vi "denso gripper.vi"() -> ()   [LabVIEW 2016]
uses:
  <vilib>/DENSO Robotics/DENSO Robot Library/_DNWA/DENSO RC8 Motion interpolation Enumeration.ctl
  <vilib>/DENSO Robotics/DENSO Robot Library/_DNWA/DENSO RC8 Motion Option Cluster.ctl
  <vilib>/DigiMetrix/Schunk WSG Library/Schunk WSG library.lvlib
  <vilib>/DENSO Robotics/DENSO Robot Library/_DNWA/RC8 Library.lvlib
panel:
  out "element":dbl
  out "array":dbl[][](array[numeric])
  in  "IP address":string="192.168.1.140"
  out "error out":errorcluster
  out "?":string
  in  "Motion interpolation":T1=1 items=["P"=1, "L"=2, "C"=3]
  out "success":bool
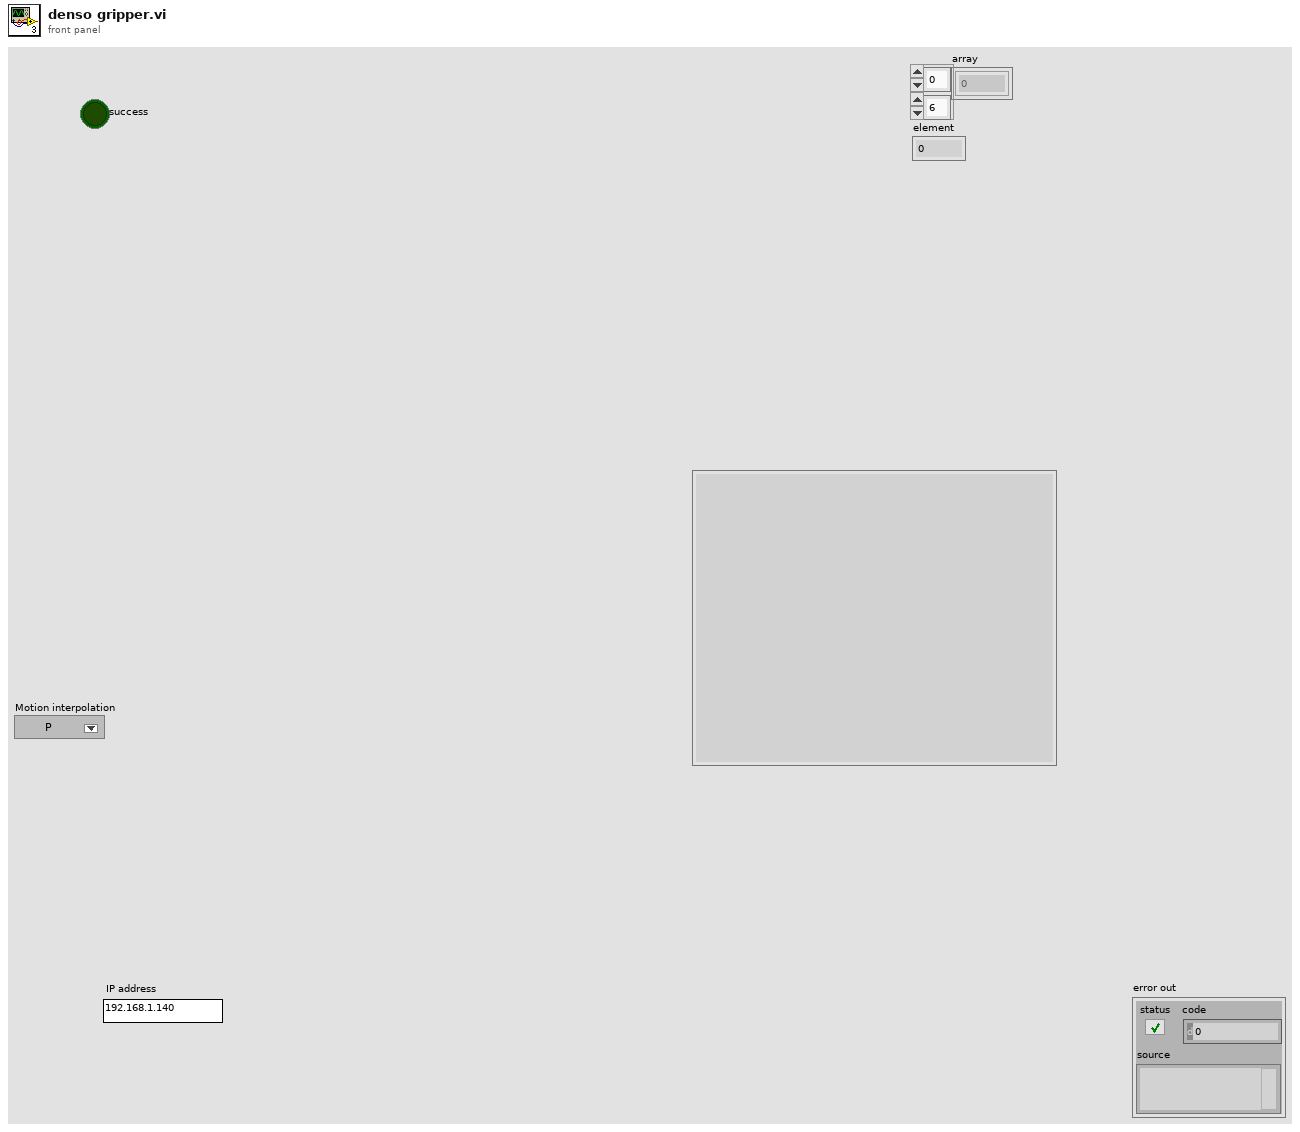
[diagram p1: front panel]
types:
  T1 = typedef "DENSO b-CAP Library.lvlib/RC8 Library.lvlib/DENSO RC8 Motion interpolation Enumeration.ctl" = i32
  T2 = typedef "DENSO b-CAP Library.lvlib/RC8 Library.lvlib/DENSO RC8 Motion Option Cluster.ctl" = cluster{"Asynchronous execution option":bool, "[SPEED=n][,ACCEL=n][,DECEL=n][,TIME=n]":string}
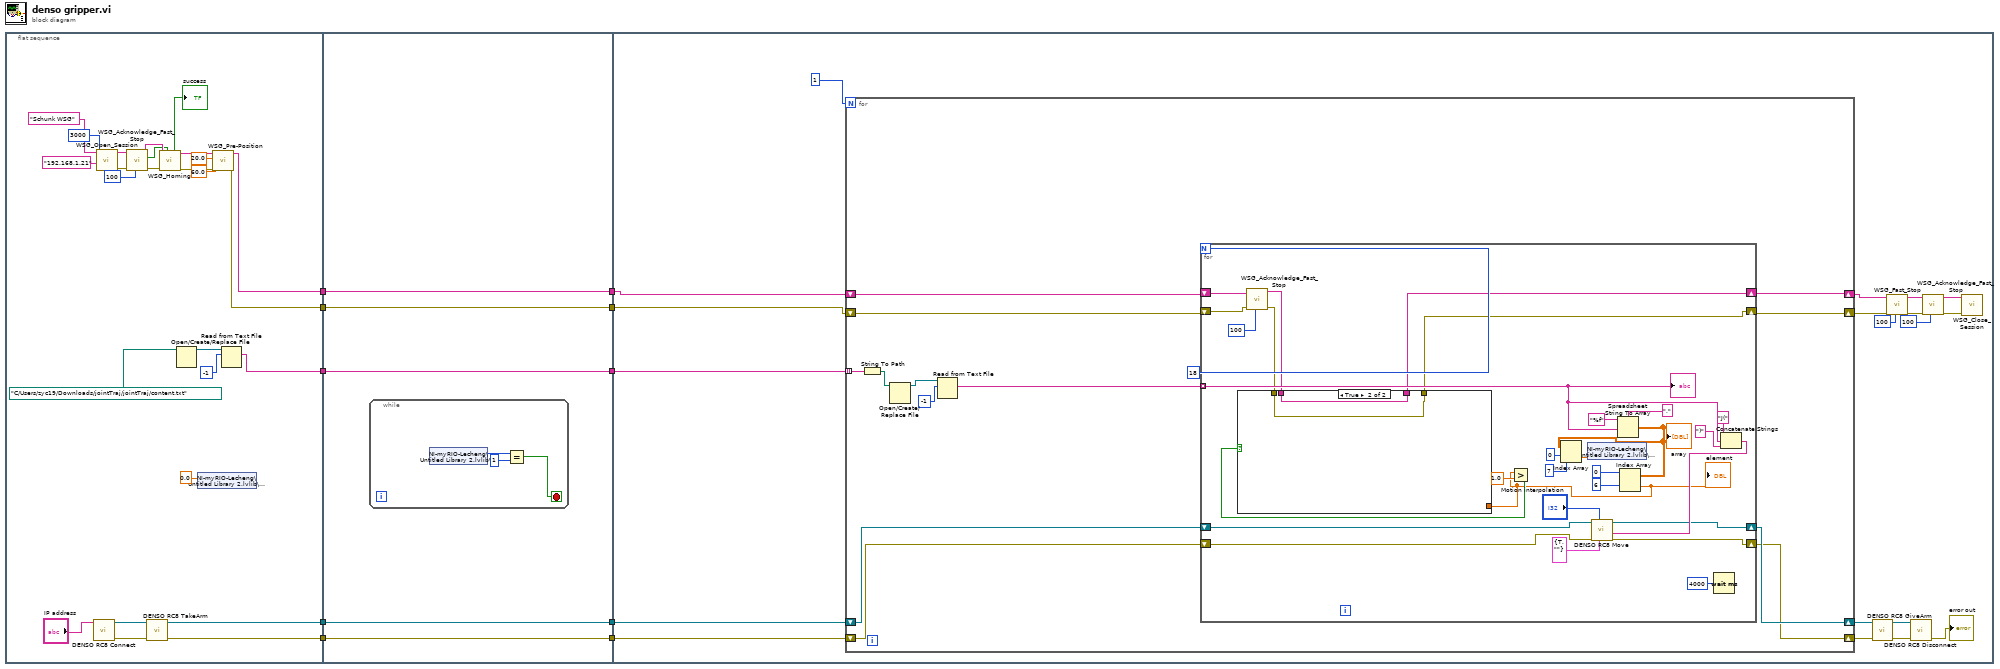
[diagram p0: block diagram]
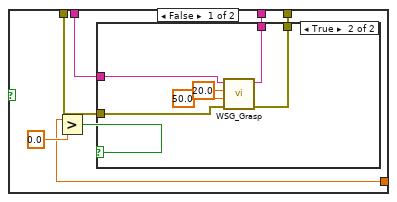
[diagram p2: hidden frame]
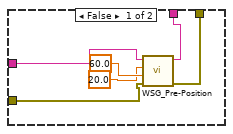
[diagram p3: hidden frame]
diagram:
  n1 = flat-sequence {
    tunnel: [w30] -> w10
    tunnel: [w29] -> w8
    tunnel: [w28] -> w5
    tunnel: [w13] -> w3
    tunnel: [w12] -> w2
    tunnel: w10 -> [w41]
    tunnel: [w41] -> w9
    tunnel: w8 -> [w40]
    tunnel: [w40] -> w7
    tunnel: [w39] -> w6
    tunnel: w5 -> [w39]
    tunnel: [w38] -> w4
    tunnel: w3 -> [w38]
    tunnel: w2 -> [w37]
    tunnel: [w37] -> w1
    tunnel: w9 -> [w52]
    tunnel: w7 -> [w51]
    tunnel: w6 -> [w50]
    tunnel: w4 -> [w49]
    tunnel: w1 -> [w48]
    frame #0 {
      n2 = call <vilib>:"DENSO RC8 Connect.vi"("IP address"="IP address") -> ("error out"=w33:errorcluster, "DENSO b-CAP Client out"=w32:refnum<class "DENSO b-CAP Client.lvclass">)  [unwired: 9 in]
      n3 = call <vilib>:"WSG_Open_Session.vi"("ip address"="192.168.1.21", "port"=u16 3000, "wsg session name"="Schunk WSG") -> ("error out"=w27:errorcluster, "wsg session name*"=w26:string)  [unwired: 7 in]
      n4 = call <vilib>:"WSG_Acknowledge_Fast_Stop.vi"("timeout"=100, "error in (no error)"=w27, "wsg session name"=w26) -> ("error out"=w22:errorcluster, "success"=w23:bool, "wsg session name*"=w24:string)  [unwired: 5 in, 1 out]
      n5 = call <vilib>:"DENSO RC8 TakeArm.vi"("error in (no error)"=w33, "DENSO b-CAP Client in"=w32) -> ("error out"=w29:errorcluster, "DENSO b-CAP Client out"=w30:refnum<class "DENSO b-CAP Client.lvclass">)  [unwired: 8 in]
      n6 = call <vilib>:"WSG_Homing.vi"("wait fin (T)"=w23, "error in (no error)"=w22, "wsg session name"=w24) -> ("error out"=w16:errorcluster, "success"=→"success":bool, "wsg session name*"=w17:string)  [unwired: 5 in, 1 out]
      n7 = Open/Create/Replace File(file path (use dialog)=path "C:/Users/zyc19/Downloads/jointTraj/jointTraj/content.txt" ("文件路径（使用对话框）")) -> (refnum out=w36:refnum<file>)  [unwired: 1 in, 6 out]
      n8 = shared-variable "NI-myRIO-Lecheng\\Untitled Library 2.lvlib\\element"(0.0 ("element")) -> ()  [unwired: 1 in, 1 out]
      n9 = call <vilib>:"WSG_Pre-Position.vi"("error in (no error)"=w16, "pre-position width"=sgl 60.0, "pre-position speed"=sgl 20.0, "wsg session name"=w17) -> ("error out"=w12:errorcluster, "wsg session name*"=w13:string)  [unwired: 5 in, 1 out]
      n10 = Read from Text File(file (use dialog)=w36, count=-1) -> (text=w28:string[])  [unwired: 1 in, 4 out]
    }
    frame #1 {
      n11 = while {
        stop <- w42 stop-if-true
        n12 = shared-variable "NI-myRIO-Lecheng\\Untitled Library 2.lvlib\\Variable"() -> (w44:i32)  [unwired: 1 in, 1 out]
        n13 = Equal?(x=w44, y=1) -> (x = y?=w42:bool)
      }
    }
    frame #2 {
      n14 = for {
        N: 1 -> [_]
        shift-right: [w77] -> w55
        shift-left: w52 -> [w71]
        shift-right: [w76] -> w54
        shift-left: w51 -> [w70]
        tunnel: w50 -> [w68] mode=indexing
        shift-right: [w65] -> w47
        shift-left: w49 -> [w67]
        shift-right: [w64] -> w46
        shift-left: w48 -> [w66]
        n15 = String To Path(string=w68) -> (path=w73:path)
        n16 = Open/Create/Replace File(file path (use dialog)=w73) -> (refnum out=w74:refnum<file>)  [unwired: 1 in, 6 out]
        n17 = Read from Text File(file (use dialog)=w74, count=-1) -> (text=w69:string[])  [unwired: 1 in, 4 out]
        n18 = for {
          N: 18 -> [_]
          shift-right: [w101] -> w77
          shift-left: w71 -> [w102]
          shift-right: [w100] -> w76
          shift-left: w70 -> [w99]
          tunnel: w69 -> [w96] mode=indexing
          shift-right: [w84] -> w65
          shift-left: w67 -> [w88]
          shift-right: [w83] -> w64
          shift-left: w66 -> [w87]
          n19 = call <vilib>:"WSG_Acknowledge_Fast_Stop.vi"("timeout"=100, "error in (no error)"=w87, "wsg session name"=w88) -> ("error out"=w85:errorcluster, "wsg session name*"=w86:string)  [unwired: 5 in, 2 out]
          n20 = Spreadsheet String To Array(delimiter (Tab)=",", format string="%f", spreadsheet string=w96) -> (array=w92:dbl[][])  [unwired: 1 in]
          "array" <- w92
          n21 = Index Array(array=w92, index (row)=0, index (col)=7 ("disabled index (col)")) -> (element=w78:dbl)
          n22 = shared-variable "NI-myRIO-Lecheng\\Untitled Library 2.lvlib\\element"(w78) -> ()  [unwired: 1 in, 1 out]
          n23 = Index Array(array=w92, index (row)=0, index (col)=6 ("disabled index (col)")) -> (element=w80:dbl)
          "element" <- w80
          n24 = Greater?(x=w80, y=1.0) -> (0:w81:bool)
          n25 = case shown="True" w81 {
            tunnel: w86 -> [w111 w127]
            tunnel: w85 -> [w110 w126]
            tunnel: [w109 w127] -> w84
            tunnel: [w108 w126] -> w83
            tunnel: w80 -> [w107 _]
            frame False {
              n26 = Greater?(x=w107, y=0.0) -> (0:w112:bool)
              n27 = case shown="True" w112 {
                tunnel: w111 -> [w117 w123]
                tunnel: w110 -> [w116 w122]
                tunnel: [w115 w121] -> w109
                tunnel: [w114 w120] -> w108
                frame False {
                  n28 = call <vilib>:"WSG_Pre-Position.vi"("error in (no error)"=w116, "pre-position width"=sgl 60.0 ("part width"), "pre-position speed"=sgl 20.0 ("grasp speed"), "wsg session name"=w117) -> ("error out"=w114:errorcluster, "wsg session name*"=w115:string)  [unwired: 5 in, 1 out]
                }
                frame True {
                  n29 = call <vilib>:"WSG_Grasp.vi"("error in (no error)"=w122, "part width"=sgl 50.0, "grasp speed"=sgl 20.0, "wsg session name"=w123) -> ("error out"=w120:errorcluster, "wsg session name*"=w121:string)  [unwired: 4 in, 2 out]
                }
              }
            }
            frame True {
            }
          }
          n30 = Wait (ms)(milliseconds to wait=u32 4000) -> ()  [unwired: 1 out]
          n31 = Concatenate Strings("J(" ("string"), w96, ")" ("string")) -> (w105:string)
          n32 = call <vilib>:"DENSO RC8 Move.vi"("Motion option"=T2 {"Asynchronous execution option"=TRUE, "[SPEED=n][,ACCEL=n][,DECEL=n][,TIME=n]"=""}, "Motion interpolation"="Motion interpolation", "error in (no error)"=w99, "Target position"=w105, "DENSO b-CAP Client in"=w102) -> ("error out"=w100:errorcluster, "DENSO b-CAP Client out"=w101:refnum<class "DENSO b-CAP Client.lvclass">)  [unwired: 5 in]
          "?" <- w96
        }
      }
      n33 = call <vilib>:"DENSO RC8 GiveArm.vi"("error in (no error)"=w54, "DENSO b-CAP Client in"=w55) -> ("error out"=w57:errorcluster, "DENSO b-CAP Client out"=w56:refnum<class "DENSO b-CAP Client.lvclass">)  [unwired: 8 in]
      n34 = call <vilib>:"WSG_Fast_Stop.vi"("timeout"=100, "error in (no error)"=w46, "wsg session name"=w47) -> ("error out"=w63:errorcluster, "wsg session name*"=w62:string)  [unwired: 5 in, 2 out]
      n35 = call <vilib>:"DENSO RC8 Disconnect.vi"("error in (no error)"=w57, "DENSO b-CAP Client in"=w56) -> ("error out"=→"error out":errorcluster)  [unwired: 9 in]
      n36 = call <vilib>:"WSG_Acknowledge_Fast_Stop.vi"("timeout"=100, "error in (no error)"=w63, "wsg session name"=w62) -> ("error out"=w60:errorcluster, "wsg session name*"=w61:string)  [unwired: 5 in, 2 out]
      n37 = call <vilib>:"WSG_Close_Session.vi"("error in (no error)"=w60, "wsg session name"=w61) -> ()  [unwired: 9 in, 1 out]
    }
  }
